vi "HB_ThreadPool.Main.vi"() -> ()   [LabVIEW 2009, in "HB_BaseClass_Examples.lvlib"]
doc: "Simple application to test the HGF_ThreadPool with a simple class."
uses:
  HB_BaseClass_Examples.lvlib
  HB_Factory/HB_Factory.lvclass
  lib.lib/HGF_LVC/HGF_BaseClasses/HGF_Factory/HGF_Factory.lvclass
  lib.lib/HGF_LVC/HGF_BaseClasses/HGF_Visitor/HGF_Visitor.lvclass
  lib.lib/HGF_LVC/HGF_BaseClasses/HGF_Timing/HGF_Timing.lvclass
  lib.lib/HGF_LVC/HGF_BaseClasses/HGF_Queue/HGF_Queue.lvclass
  HB_Simple/HB_Simple.lvclass
  lib.lib/HGF_LVC/HGF_BaseClasses/HGF_TaskOnce/HGF_TaskOnce.lvclass
  lib.lib/HGF_LVC/HGF_BaseClasses/HGF_ThreadPool/HGF_ThreadPool.lvclass
  lib.lib/HGF_LVC/HGF_BaseClasses/HGF_Reference/HGF_Reference.lvclass
  lib.lib/HGF_LVC/HGF_BaseClasses/HGF_ThreadTask/HGF_ThreadTask.lvclass
  lib.lib/HGF_LVC/HGF_BaseClasses/HGF_Event/HGF_Event.lvclass
  lib.lib/HGF_LVC/HGF_Auxiliary/HGF_Auxiliary.lvlib
panel:
  in  "timeout in ms (-1)":i32=3000
  in  "default Destination?":bool
  out "nofTasksInQueueOut":i32
  out "nofTasksWaiting":i32
  out "autoIncrementLimit":i32=-1
  out "nofThreads":i32
  out "Monitor Loop":i32
  out "Destination timed out":bool
  out "Default Destination timed out?":bool
  out "got object?":bool
  out "error":errorcluster
  in  "Execute":bool
  in  "stop":bool
  out "values":dbl[](graph)
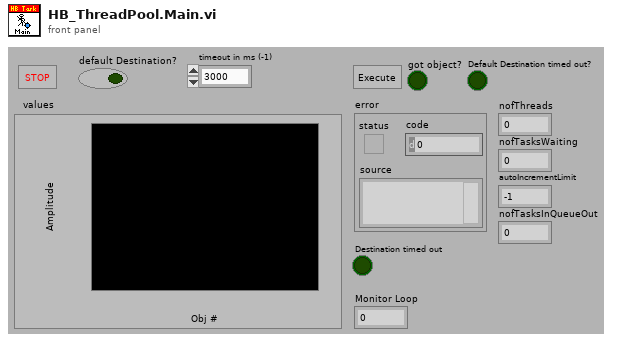
[diagram p1: front panel]
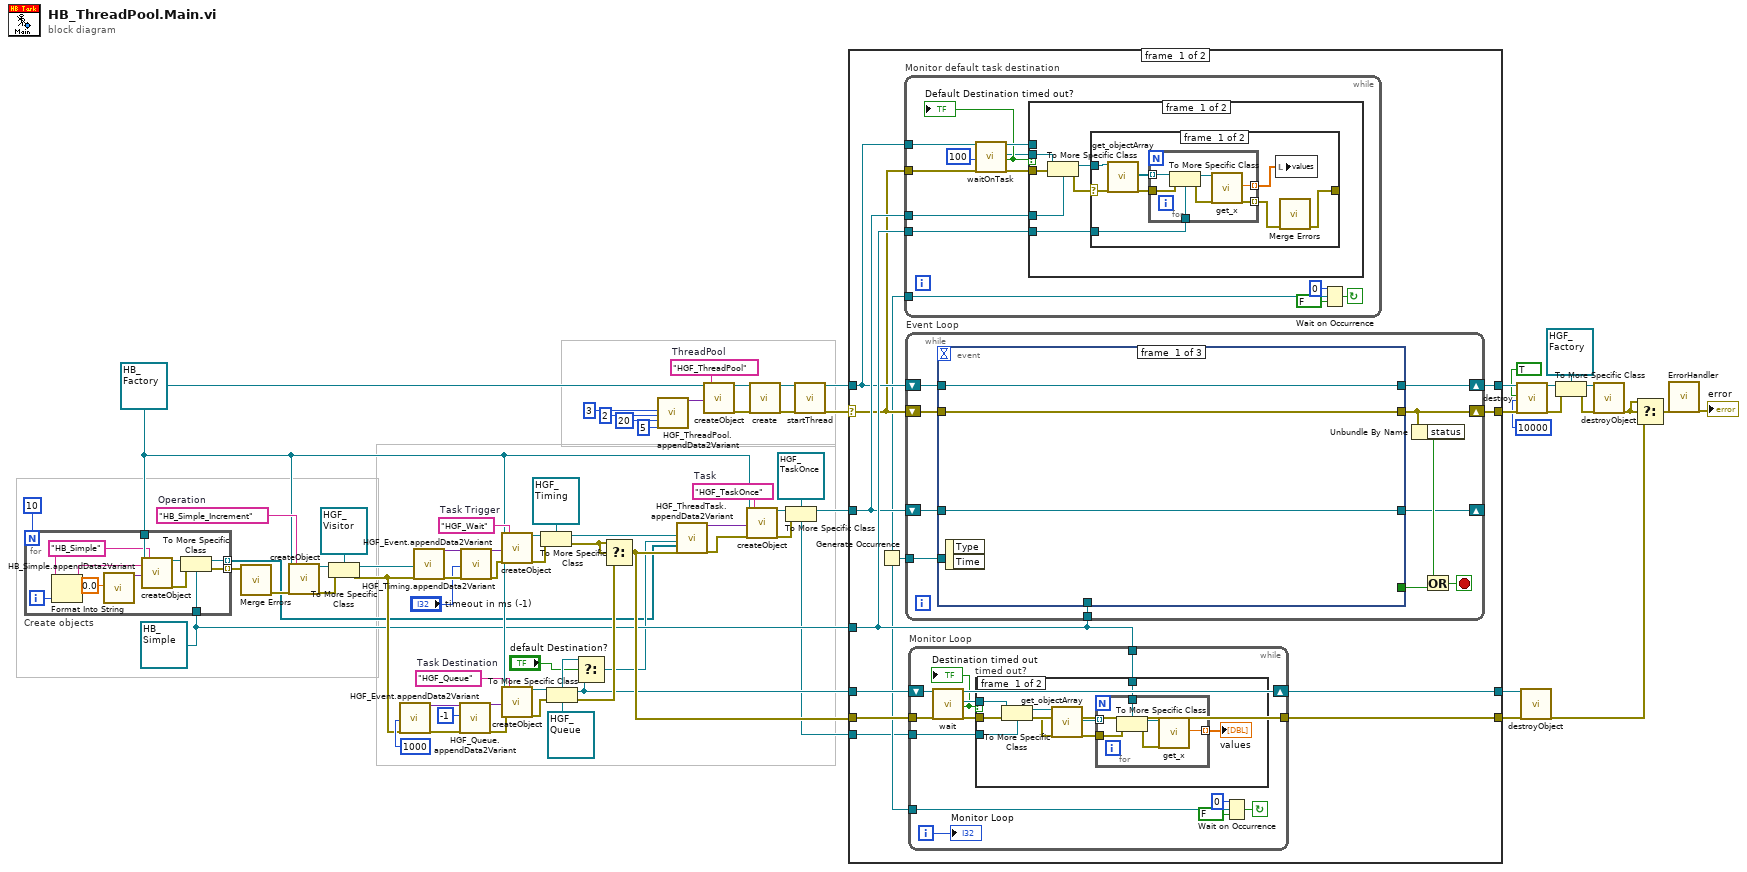
[diagram p0: block diagram]
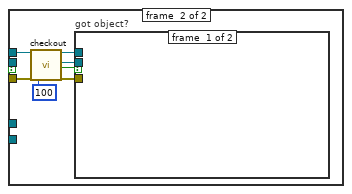
[diagram p3: hidden frame]
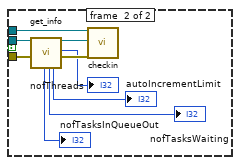
[diagram p4: hidden frame]
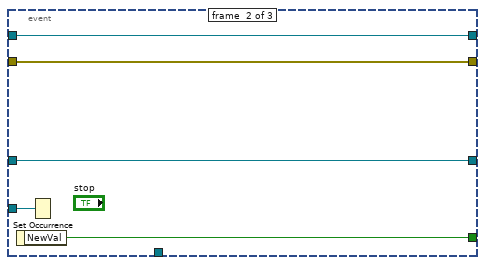
[diagram p6: hidden frame]
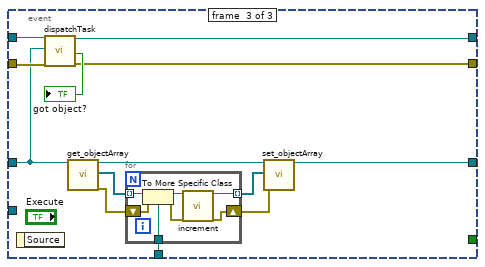
[diagram p7: hidden frame]
diagram:
  w4 = refnum<class "HGF_TaskOnce.lvclass"> refnum ("HGF_BaseClasses.lvlib:HGF_ThreadTaskOnce.lvclass")
  w12 = refnum<class "HB_Simple.lvclass"> refnum ("HB_Simple.lvclass")
  w10 = "HGF_Queue"  # Task Destination
  w9 = refnum<class "HGF_Queue.lvclass"> refnum ("HGF_BaseClasses.lvlib:HGF_Queue.lvclass")
  w43 = "HB_Simple_Increment"  # Operation
  w42 = "HGF_Wait"  # Task Trigger
  w41 = "HGF_TaskOnce"  # Task
  w11 = "HGF_ThreadPool"  # ThreadPool
  w35 = refnum<class "HB_Factory.lvclass"> refnum ("HB_Factory.lvclass")
  n1 = for "Create objects" {
    N: 10 -> [_]
    tunnel: w35 -> [w82]
    tunnel: [w79] -> w1 mode=indexing
    tunnel: [w78] -> w53 mode=indexing
    tunnel: w12 -> [w73]
    i -> [w77]
    w76 = "HB_Simple" ("className")
    n2 = Format Into String(initial string=w76, w77) -> (resulting string=w75:string)  [unwired: 2 in, 1 out]
    n3 = call "HB_Simple.appendData2Variant.vi"("x"=0.0) -> ("dup initData"=w81:variant)  [unwired: 17 in, 1 out]
    n4 = call "createObject.vi"("HGF_Factory"=w82, "objectName"=w75, "initializationData"=w81, "className"=w76) -> ("HGF_Object"=w74:refnum<class "HGF_Factory.lvclass">, "error out"=w83:errorcluster)  [unwired: 2 in, 12 out]
    n5 = To More Specific Class(target class=w73, reference=w74, error in=w83) -> (specific class reference=w79:refnum<class "HB_Simple.lvclass">, error out=w78:errorcluster)
  }
  n6 = call <vilib>:"Merge Errors.vi"("error array in"=w53) -> ("error out"=w17:errorcluster)  [unwired: 3 in, 3 out]
  n7 = call "createObject.vi"("HGF_Factory"=w35, "error in (no error)"=w17, "className"=w43) -> ("HGF_Object"=w39:refnum<class "HGF_Factory.lvclass">, "error out"=w38:errorcluster)  [unwired: 3 in, 12 out]
  n8 = To More Specific Class(target class=refnum<class "HGF_Visitor.lvclass"> refnum ("HGF_BaseClasses.lvlib:HGF_Visitor.lvclass"), reference=w39, error in=w38) -> (specific class reference=w46:refnum<class "HGF_Visitor.lvclass">, error out=w16:errorcluster)
  n9 = call "HGF_Event.appendData2Variant.vi"("timeout in ms (-1)"=1000, "error in (no error)"=w16) -> ("dup initData"=w29:variant, "error out"=w30:errorcluster)  [unwired: 2 in, 14 out]
  n10 = call "HGF_Timing.appendData2Variant.vi"("defaultObject"=w46, "error in (no error)"=w16) -> ("dup initData"=w47:variant, "error out"=w45:errorcluster)  [unwired: 1 in, 15 out]
  n11 = call "HGF_Queue.appendData2Variant.vi"("initData"=w29, "maxQueueSize (-1)"=-1, "error in (no error)"=w30) -> ("dup initData"=w31:variant, "error out"=w32:errorcluster)  [unwired: 15 out]
  n12 = call "HGF_Event.appendData2Variant.vi"("initData"=w47, "timeout in ms (-1)"="timeout in ms (-1)", "error in (no error)"=w45) -> ("dup initData"=w57:variant, "error out"=w56:errorcluster)  [unwired: 1 in, 14 out]
  n13 = call "createObject.vi"("HGF_Factory"=w35, "initializationData"=w57, "error in (no error)"=w56, "className"=w42) -> ("HGF_Object"=w37:refnum<class "HGF_Factory.lvclass">, "error out"=w58:errorcluster)  [unwired: 2 in, 12 out]
  n14 = call "createObject.vi"("HGF_Factory"=w35, "initializationData"=w31, "error in (no error)"=w32, "className"=w10) -> ("HGF_Object"=w34:refnum<class "HGF_Factory.lvclass">, "error out"=w33:errorcluster)  [unwired: 2 in, 12 out]
  n15 = To More Specific Class(target class=refnum<class "HGF_Timing.lvclass"> refnum ("HGF_BaseClasses.lvlib:HGF_Timing.lvclass"), reference=w37, error in=w58) -> (specific class reference=w59:refnum<class "HGF_Timing.lvclass">, error out=w15:errorcluster)
  n16 = To More Specific Class(target class=w9, reference=w34, error in=w33) -> (specific class reference=w8:refnum<class "HGF_Queue.lvclass">, error out=w14:errorcluster)
  n17 = Select(t=w9, s="default Destination?", f=w8) -> (s? t:f=w7:refnum<class "HGF_Queue.lvclass">)
  n18 = Select(t=w15, s=w15, f=w14) -> (s? t:f=w13:errorcluster)
  n19 = call "HGF_ThreadPool.appendData2Variant.vi"("initialNofThreads (0)"=3 ("initialNofThreads"), "incThreads(1)"=2 ("incThreads"), "maxNofThreads (-1:unlimited)"=20 ("maxNofThreads"), "autoIncrementLimit (-1)"=5) -> ("dup initData"=w71:variant)  [unwired: 3 in, 12 out]
  n20 = call "HGF_ThreadTask.appendData2Variant.vi"("taskTrigger"=w59, "taskDestination"=w7, "objectArray"=w1, "error in (no error)"=w13) -> ("dup initData"=w3:variant, "error out"=w2:errorcluster)  [unwired: 2 in, 12 out]
  n21 = call "createObject.vi"("HGF_Factory"=w35, "initializationData"=w71, "className"=w11) -> ("HGF_Object"=w40:refnum<class "HGF_Factory.lvclass">, "error out"=w70:errorcluster)  [unwired: 3 in, 12 out]
  n22 = call "createObject.vi"("HGF_Factory"=w35, "initializationData"=w3, "error in (no error)"=w2, "className"=w41) -> ("HGF_Object"=w36:refnum<class "HGF_Factory.lvclass">, "error out"=w52:errorcluster)  [unwired: 2 in, 12 out]
  n23 = call "create.vi"("Object"=w40, "error in (no error)"=w70) -> ("HGF_Reference"=w72:refnum<class "HGF_Reference.lvclass">, "error out"=w66:errorcluster)  [unwired: 1 in, 15 out]
  n24 = To More Specific Class(target class=w4, reference=w36, error in=w52) -> (specific class reference=w50:refnum<class "HGF_TaskOnce.lvclass">)  [unwired: 1 out]
  n25 = call "startThread.vi"("HGF_ThreadPool_Reference"=w72, "error in (no error)"=w66) -> ("dup HGF_ThreadPool_Reference"=w60:refnum<class "HGF_Reference.lvclass">, "error out"=w48:errorcluster)  [unwired: 1 in, 15 out]
  n26 = case shown="No Error" w48 {
    selector: w48 -> [w86 w216]
    tunnel: w60 -> [w87 w217]
    tunnel: [w95 w217] -> w51
    tunnel: w50 -> [w88 _]
    tunnel: [w94 w216] -> w49
    tunnel: w8 -> [w93 w215]
    tunnel: [w92 w215] -> w26
    tunnel: w13 -> [w91 w214]
    tunnel: [w90 w214] -> w21
    tunnel: w12 -> [w89 _]
    tunnel: w4 -> [w84 _]
    frame #0 {
      n27 = Generate Occurrence() -> (w85:refnum<k4>)
      n28 = while "Monitor default task destination" {
        tunnel: w89 -> [w104]
        tunnel: w88 -> [w103]
        tunnel: w87 -> [w102]
        tunnel: w86 -> [w101]
        tunnel: w85 -> [w96]
        stop <- w97 continue-if-true
        n29 = call "waitOnTask.vi"("HGF_ThreadPool_Reference"=w102, "timeout in ms (-1)"=100, "error in (no error)"=w101) -> ("dup HGF_ThreadPool_Reference"=w108:refnum<class "HGF_Reference.lvclass">, "HGF_Task"=w106:refnum<class "HGF_ThreadTask.lvclass">, "timed out?"=w107:bool, "error out"=w100:errorcluster)  [unwired: 13 out]
        "Default Destination timed out?" <- w107
        n30 = case "timed out?" shown="False" w107 {
          tunnel: w106 -> [w114 _]
          tunnel: w100 -> [w113 w131]
          tunnel: w108 -> [_ w132]
          tunnel: w104 -> [w110 _]
          tunnel: w103 -> [w109 _]
          frame #0 {
            n31 = To More Specific Class(target class=w109, reference=w114, error in=w113) -> (specific class reference=w112:refnum<class "HGF_TaskOnce.lvclass">, error out=w111:errorcluster)
            n32 = case shown="No Error" w111 {
              selector: w111 -> [w121 w130]
              tunnel: w112 -> [w122 _]
              tunnel: [w117 w130] -> _
              tunnel: w110 -> [w115 _]
              frame #0 {
                n33 = call "get_objectArray.vi"("HGF_ThreadTask"=w122, "error in (no error)"=w121) -> ("objectArray"=w120:refnum<class>[], "error out"=w116:errorcluster)  [unwired: 16 out]
                n34 = for {
                  tunnel: w116 -> [w128]
                  tunnel: [w125] -> _ mode=indexing
                  tunnel: [w126] -> w119 mode=indexing
                  tunnel: w120 -> [w125] mode=indexing
                  tunnel: [w124] -> w118 mode=indexing
                  tunnel: w115 -> [w123]
                  n35 = To More Specific Class(target class=w123, reference=w125, error in=w128) -> (specific class reference=w129:refnum<class "HB_Simple.lvclass">, error out=w127:errorcluster)
                  n36 = call "get_x.vi"("HB_Simple"=w129, "error in (no error)"=w127) -> ("x"=w126:dbl, "error out"=w124:errorcluster)  [unwired: 16 out]
                }
                n37 = local write "values"(w119) -> ()
                n38 = call <vilib>:"Merge Errors.vi"("error array in"=w118) -> ("error out"=w117:errorcluster)  [unwired: 3 in, 3 out]
              }
              frame #1 {
              }
            }
          }
          frame #1 {
            n39 = call "checkout.vi"("HGF_ThreadPool_Reference"=w132, "timeout in ms (-1)"=100, "error in (no error)"=w131) -> ("dup HGF_ThreadPool_Reference"=w133:refnum<class "HGF_Reference.lvclass">, "HGF_ThreadPool"=w134:refnum<class "HGF_ThreadPool.lvclass">, "got object?"=w137:bool, "error out"=w135:errorcluster)  [unwired: 13 out]
            n40 = case "got object?" shown="True" w137 {
              tunnel: w133 -> [_ w146]
              tunnel: w134 -> [_ w145]
              tunnel: w135 -> [_ w144]
              frame #0 {
              }
              frame #1 {
                n41 = call "get_info.vi"("HGF_ThreadPool"=w145, "error in (no error)"=w144) -> ("nofTasksInQueueOut"=→"nofTasksInQueueOut":i32, "nofTasksWaiting"=→"nofTasksWaiting":i32, "autoIncrementLimit"=→"autoIncrementLimit":i32, "dup HGF_ThreadPool"=w142:refnum<class "HGF_ThreadPool.lvclass">, "nofThreads"=→"nofThreads":i32, "error out"=w143:errorcluster)  [unwired: 12 out]
                n42 = call "checkin.vi"("HGF_Reference"=w146, "Object"=w142, "error in (no error)"=w143) -> ()  [unwired: 1 in, 16 out]
              }
            }
          }
        }
        n43 = Wait on Occurrence(1:FALSE ("ignore previous (T)"), 2:w96, 3:0 ("ms timeout (-1)")) -> (0:w97:bool)
      }
      n44 = while "Event Loop" {
        tunnel: w89 -> [w175]
        shift-right: [w176] -> _
        shift-left: w88 -> [w177]
        shift-right: [w179] -> w95
        shift-left: w87 -> [w178]
        tunnel: w85 -> [w183]
        shift-right: [w181] -> w94
        shift-left: w86 -> [w180]
        stop <- w185 stop-if-true
        n45 = event shown="[2] \"Execute\": Value Change" {
          selector: _ -> [_ _ _]
          dyn-events: _ -> [_ _ _]
          timeout: _ -> [_ _ _]
          tunnel: w183 -> [_ w193 _]
          tunnel: [_ w192 _] -> w182
          tunnel: [w187 w191 w194] -> w181
          tunnel: w180 -> [w187 w191 w205]
          tunnel: [w188 w190 w195] -> w179
          tunnel: w178 -> [w188 w190 w206]
          tunnel: w177 -> [w186 w189 w199]
          tunnel: [w186 w189 w197] -> w176
          tunnel: w175 -> [_ _ w196]
          event #0 {
            n46 = event-data() -> ()  [unwired: 3 out]
          }
          event #1 {
            n47 = event-data() -> ("NewVal"=w192:bool)  [unwired: 1 out]
            n48 = Set Occurrence(w193) -> ()
          }
          event #2 {
            n49 = event-data() -> ()  [unwired: 2 out]
            n50 = call "dispatchTask.vi"("HGF_ThreadPool_Reference"=w206, "HGF_ThreadTask"=w199, "error in (no error)"=w205) -> ("dup HGF_ThreadPool_Reference"=w195:refnum<class "HGF_Reference.lvclass">, "got object?"=→"got object?":bool, "error out"=w194:errorcluster)  [unwired: 1 in, 13 out]
            n51 = call "get_objectArray.vi"("HGF_ThreadTask"=w199) -> ("dup HGF_ThreadTask"=w198:refnum<class "HGF_TaskOnce.lvclass">, "objectArray"=w200:refnum<class>[], "error out"=w201:errorcluster)  [unwired: 1 in, 15 out]
            n52 = for {
              tunnel: w200 -> [w213] mode=indexing
              tunnel: [w209] -> w202 mode=indexing
              shift-right: [w208] -> w203
              shift-left: w201 -> [w212]
              tunnel: w196 -> [w207]
              n53 = To More Specific Class(target class=w207, reference=w213, error in=w212) -> (specific class reference=w210:refnum<class "HB_Simple.lvclass">, error out=w211:errorcluster)
              n54 = call "increment.vi"("HB_Simple in"=w210, "error in (no error)"=w211) -> ("HB_Simple out"=w209:refnum<class "HB_Simple.lvclass">, "error out"=w208:errorcluster)  [unwired: 16 out]
            }
            n55 = call "set_objectArray.vi"("HGF_ThreadTask"=w198, "objectArray"=w202, "error in (no error)"=w203) -> ("dup HGF_ThreadTask"=w197:refnum<class "HGF_TaskOnce.lvclass">)  [unwired: 1 in, 15 out]
          }
        }
        n56 = Unbundle By Name(w181) -> ("status"=w184:bool)
        n57 = Or(x=w184, y=w182) -> (x .or. y?=w185:bool)
      }
      n58 = while "Monitor Loop" {
        shift-right: [w157] -> w92
        shift-left: w93 -> [w159]
        tunnel: w91 -> [w156]
        tunnel: w85 -> [w153]
        tunnel: w89 -> [w151]
        tunnel: [w149] -> w90
        tunnel: w84 -> [w147]
        i -> [w148]
        stop <- w155 continue-if-true
        n59 = call-dynamic "wait.vi"("HGF_Queue"=w159, "error in (no error)"=w156) -> ("dup HGF_Queue"=w157:refnum<class "HGF_Queue.lvclass">, "Object"=w158:refnum<class>, "timed out"=w150:bool, "error out"=w149:errorcluster)  [unwired: 2 in, 12 out]
        "Destination timed out" <- w150
        n60 = case "timed out?" shown="False" w150 {
          tunnel: w149 -> [w168 _]
          tunnel: w158 -> [w167 _]
          tunnel: w151 -> [w162 _]
          tunnel: w147 -> [w161 _]
          frame #0 {
            n61 = To More Specific Class(target class=w161, reference=w167, error in=w168) -> (specific class reference=w163:refnum<class "HGF_TaskOnce.lvclass">, error out=w160:errorcluster)
            n62 = call "get_objectArray.vi"("HGF_ThreadTask"=w163, "error in (no error)"=w160) -> ("objectArray"=w165:refnum<class>[], "error out"=w164:errorcluster)  [unwired: 16 out]
            n63 = for {
              tunnel: w164 -> [w172]
              tunnel: w165 -> [w174] mode=indexing
              tunnel: [w170] -> w166 mode=indexing
              tunnel: w162 -> [w169]
              n64 = To More Specific Class(target class=w169, reference=w174, error in=w172) -> (specific class reference=w173:refnum<class "HB_Simple.lvclass">, error out=w171:errorcluster)
              n65 = call "get_x.vi"("HB_Simple"=w173, "error in (no error)"=w171) -> ("x"=w170:dbl)  [unwired: 17 out]
            }
            "values" <- w166
          }
          frame #1 {
          }
        }
        n66 = Wait on Occurrence(1:FALSE ("ignore previous (T)"), 2:w153, 3:0 ("ms timeout (-1)")) -> (0:w155:bool)
        "Monitor Loop" <- w148
      }
    }
    frame #1 {
    }
  }
  n67 = call "destroy.vi"("HGF_Reference"=w51, "wait for activity? (F)"=TRUE, "timeout /ms (-1)"=10000, "error in (no error)"=w49) -> ("Object"=w65:refnum<class>, "error out"=w63:errorcluster)  [unwired: 14 out]
  n68 = call "destroyObject.vi"("HGF_Factory"=w26, "error in (no error)"=w21) -> ("error out"=w25:errorcluster)  [unwired: 17 out]
  n69 = To More Specific Class(target class=refnum<class "HGF_Factory.lvclass"> refnum ("HGF_BaseClasses.lvlib:HGF_Factory.lvclass"), reference=w65, error in=w63) -> (specific class reference=w64:refnum<class "HGF_Factory.lvclass">, error out=w62:errorcluster)
  n70 = call "destroyObject.vi"("HGF_Factory"=w64, "error in (no error)"=w62) -> ("error out"=w24:errorcluster)  [unwired: 17 out]
  n71 = Select(t=w24, s=w24, f=w25) -> (s? t:f=w23:errorcluster)
  n72 = call "ErrorHandler.vi"("error in (no error)"=w23) -> ("error out"=→"error":errorcluster)  [unwired: 6 in, 12 out]
